vi "Result_Test.vi"(8 "error in (no error)":errorcluster caption="entrée d'erreur (pas d'erreur)", 11 "Flash_Jlink en entrée":refnum<class "Nodon_ZCR_Delta_OFF.lvclass">) -> (0 "error out":errorcluster caption="sortie d'erreur", 3 "Flash_Jlink en sortie":refnum<class "Nodon_ZCR_Delta_OFF.lvclass">)   [LabVIEW 2020, in "Library Test.lvlib" / "Nodon_ZCR_Delta_OFF.lvclass"]
uses:
  Nodon_ZCR_Delta_OFF.lvclass
  C:/Users/ngarcin/OneDrive - Altyor/Standard TB/Suite TB45/Class/Test/Test (Default)/Test (Default).lvclass
  Commun VI/TypeDef/Variable Printable.ctl
  Test_Without_Instr/Test_Without_Inst.lvclass
  Commun VI/Library Commun.lvlib
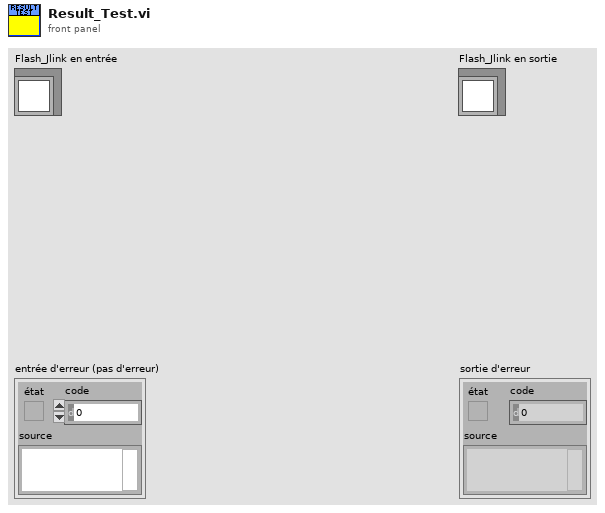
[diagram p1: front panel]
types:
  T1 = cluster{"Décallage sinus On":dbl, "Décallage sinus Off":dbl}
  T2 = typedef "Variable Printable.ctl" = string
  T3 = enum16{"Get Variable", "Get All Variables", "Set Variable", "Delete Variable", "Delete All Variable"}
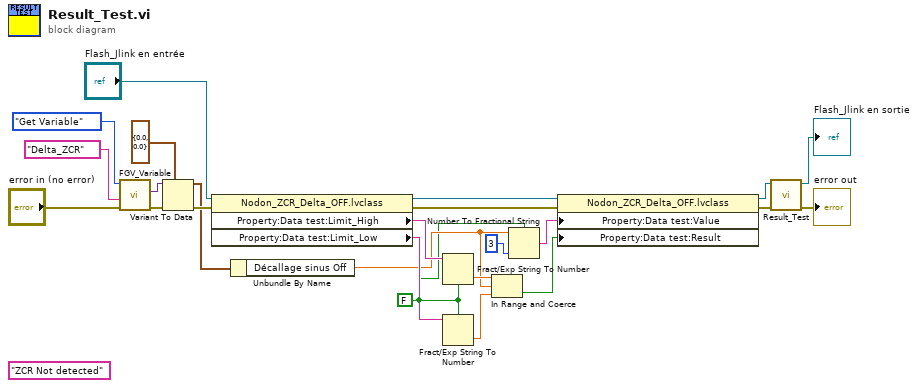
[diagram p0: block diagram]
diagram:
  (unwired) "ZCR Not detected" ("cas faux")
  w1 = FALSE ("utiliser le séparateur décimal du système (V)")
  n1 = call "FGV_Variable.vi"("error in (no error)"="error in (no error)", "Variable"=T2 "Delta_ZCR", "Function"=T3."Get Variable") -> ("error out"=w16:errorcluster, "Data Out"=w15:variant)  [unwired: 6 in, 1 out]
  n2 = Variant To Data(error in=w16, type=T1 {"Décallage sinus On"=0.0, "Décallage sinus Off"=0.0} ("Controle Decalage"), Variant=w15) -> (data=w4:T1, error out=w9:errorcluster)
  n3 = property class="Nodon_ZCR_Delta_OFF.lvclass"(reference="Flash_Jlink en entrée", error in=w9) -> (reference out=w6:refnum<class "Nodon_ZCR_Delta_OFF.lvclass">, error out=w7:errorcluster, "Property:Data test:Limit_High"=w10:string, "Property:Data test:Limit_Low"=w5:string)
  n4 = Unbundle By Name(w4) -> ("Décallage sinus Off"=w3:dbl)
  n5 = Fract/Exp String To Number(use system decimal point (T)=w1, string=w10) -> (number=w13:dbl)  [unwired: 2 in, 1 out]
  n6 = Fract/Exp String To Number(use system decimal point (T)=w1, string=w5) -> (number=w12:dbl)  [unwired: 2 in, 1 out]
  n7 = In Range and Coerce(upper limit=w13, x=w3, lower limit=w12) -> (In Range?=w2:bool)  [unwired: 1 out]
  n8 = Number To Fractional String(use system decimal point (T)=w1, number=w3, precision (6)=i16 3 ("précision (6)")) -> (F-format string=w20:string)  [unwired: 1 in]
  n9 = property class="Nodon_ZCR_Delta_OFF.lvclass"(reference=w6, error in=w7, "Property:Data test:Value"=w20, "Property:Data test:Result"=w2) -> (reference out=w21:refnum<class "Nodon_ZCR_Delta_OFF.lvclass">, error out=w22:errorcluster)
  n10 = call-parent "Result_Test.vi"("error in (no error)"=w22, "Test_Without_Inst en entrée"=w21) -> ("error out"=→"error out":errorcluster, "Test_Without_Inst en sortie"=→"Flash_Jlink en sortie":refnum<class "Nodon_ZCR_Delta_OFF.lvclass">)  [unwired: 8 in]
